vi "Update Set Defaults.vi"(4 "Project Ref":refnum<vi>, 6 "Names":string[](array[string]), 7 "Entity Paths":T1, 8 "error in (no error)":errorcluster) -> (0 "error":errorcluster)   [LabVIEW 2020, in "Conditum-Tools.lvlib" / "Entity Editor.lvclass"]
uses:
  Entity Editor.lvclass
  Entity Paths.ctl
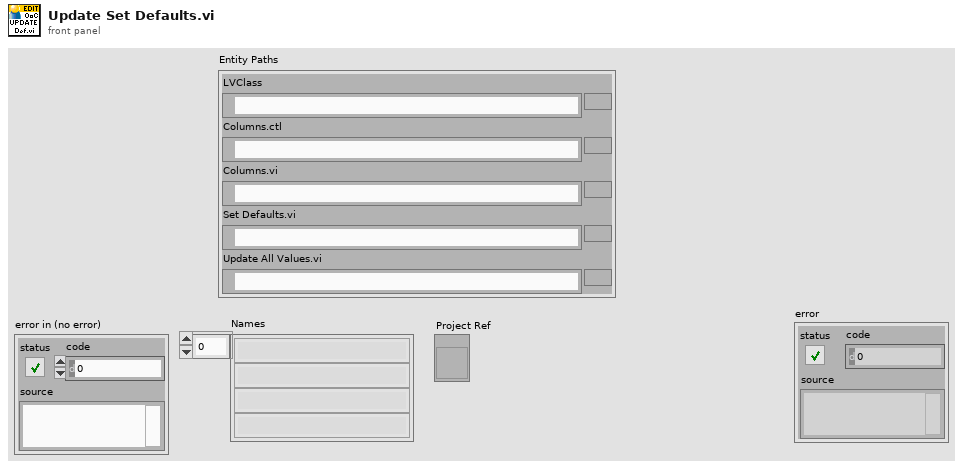
[diagram p1: front panel]
types:
  T1 = typedef "Conditum-Tools.lvlib/Entity Editor.lvclass/Entity Paths.ctl" = cluster{"LVClass":path, "Columns.ctl":path, "Columns.vi":path, "Set Defaults.vi":path, "Update All Values.vi":path}
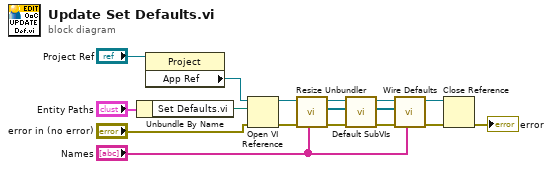
[diagram p0: block diagram]
diagram:
  n1 = Unbundle By Name("Entity Paths") -> ("Set Defaults.vi"=w16:path)
  n2 = property class="Project"(reference="Project Ref") -> ("App Ref"=w14:refnum<vi>)  [unwired: 1 in, 2 out]
  n3 = Open VI Reference(application reference (local)=w14, vi path=w16, error in (no error)="error in (no error)") -> (vi reference=w10:refnum<vi>, error out=w11:errorcluster)  [unwired: 3 in]
  n4 = call "Resize Unbundler.vi"("Names"="Names", "error in (no error)"=w11, "VI in"=w10) -> ("error out"=w8:errorcluster, "Unbundler Terminals"=w7:refnum<vi>[], "VI"=w9:refnum<vi>)  [unwired: 6 in]
  n5 = call "Default SubVIs.vi"("error in (no error)"=w8, "Unbundler Terminals"=w7, "VI in"=w9) -> ("error out"=w6:errorcluster, "SubVI Outputs"=w4:refnum<vi>[], "VI"=w5:refnum<vi>)  [unwired: 6 in]
  n6 = call "Wire Defaults.vi"("Names"="Names", "error in (no error)"=w6, "SubVI Outputs"=w4, "VI in"=w5) -> ("error out"=w3:errorcluster, "VI"=w2:refnum<vi>)  [unwired: 6 in]
  n7 = Close Reference(reference=w2, error in (no error)=w3) -> (error out=→"error":errorcluster)
